vi "SFP Calculate Column Widths for Info Table.vi"(8 "minimum width":u32=4, 9 "default width":u32=236, 10 "number of columns":i32=3, 11 "total width":u32=800) -> (3 "column widths":u32[](array[numeric]))   [LabVIEW 2017]
doc: "given a total width and number of columns, this VI calculates the column width for each column to that column widths are default width if possible, minimum width as necessary, and the first column expands to fill remaining space."
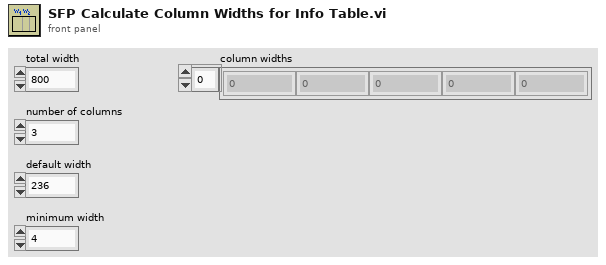
[diagram p1: front panel]
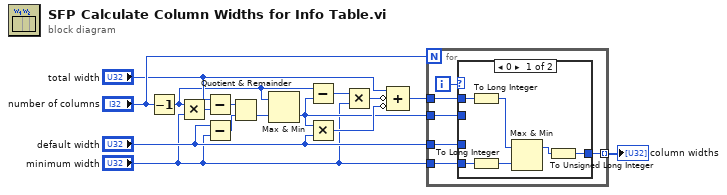
[diagram p0: block diagram]
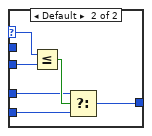
[diagram p2: hidden frame]
diagram:
  n1 = Decrement(x="number of columns") -> (x-1=w4:i32)
  n2 = Multiply(x=w4, y="minimum width") -> (x*y=w13:u32)
  n3 = Subtract(x="total width", y=w13) -> (x-y=w14:u32)
  n4 = Subtract(x="default width", y="minimum width") -> (x-y=w15:u32)
  n5 = Quotient & Remainder(x=w14, y=w15) -> (floor(x/y)=w3:u32)  [unwired: 1 out]
  n6 = Max & Min(x=w4, y=w3) -> (min(x,y)=w2:u32)  [unwired: 1 out]
  n7 = Subtract(x=w4, y=w2) -> (x-y=w11:u32)
  n8 = Multiply(x=w2, y="default width") -> (x*y=w8:u32)
  n9 = Multiply(x=w11, y="minimum width") -> (x*y=w9:u32)
  n10 = Compound Arithmetic op=ADD("total width", invert w9, invert w8) -> (w7:u32)
  n11 = for {
    N: "number of columns" -> [_]
    tunnel: w7 -> [w20]
    tunnel: [w19] -> w5 mode=indexing
    tunnel: w2 -> [w18]
    tunnel: "default width" -> [w17]
    tunnel: "minimum width" -> [w16]
    i -> [w21]
    n12 = case shown="0" w21 {
      selector: w21 -> [_ w31]
      tunnel: w20 -> [w27 _]
      tunnel: [w23 w33] -> w19
      tunnel: w18 -> [_ w30]
      tunnel: w17 -> [_ w29]
      tunnel: w16 -> [w22 w28]
      frame 0 {
        n13 = To Long Integer(number=w27) -> (32bit integer=w26:i32)
        n14 = To Long Integer(number=w22) -> (32bit integer=w25:i32)
        n15 = Max & Min(x=w26, y=w25) -> (max(x,y)=w24:i32)  [unwired: 1 out]
        n16 = To Unsigned Long Integer(number=w24) -> (unsigned 32bit integer=w23:u32)
      }
      frame Default {
        n17 = Less Or Equal?(x=w31, y=w30) -> (x <= y?=w32:bool)
        n18 = Select(t=w29, s=w32, f=w28) -> (s? t:f=w33:u32)
      }
    }
  }
  "column widths" <- w5
